vi "Read SubComponents.vi"(8 "error in (no error)":errorcluster, 11 "1553 Component in":refnum<class "1553 Component.lvclass">) -> (0 "error out":errorcluster, 2 "SubComponents":refnum<class "1553 SubComponent.lvclass">[](array[class]), 3 "1553 Component out":refnum<class "1553 Component.lvclass">)   [LabVIEW 2020, in "BCI-1553 API.lvlib" / "1553 Component.lvclass"]
doc: "Returns all the subcomponents being used by this component in a 1553 Session. After initialization, where applicable, all subcomponents are returned in this order:\n\n0: Bus Controller\n1-2: Remote Terminal(s)\n3: Bus Monitor\n\nThe order shifts towards index 0 if a subcomponent is not present during the initialization."
uses:
  1553 Component.lvclass
  1553 SubComponent/1553 SubComponent.lvclass
  1553 Component.lvclass/1553 Component.ctl
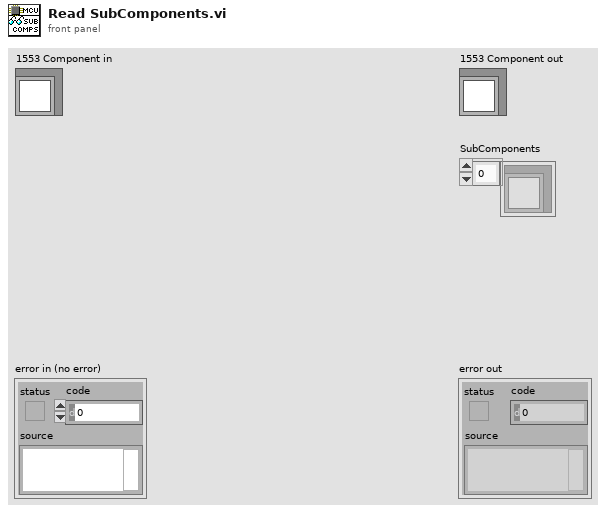
[diagram p1: front panel]
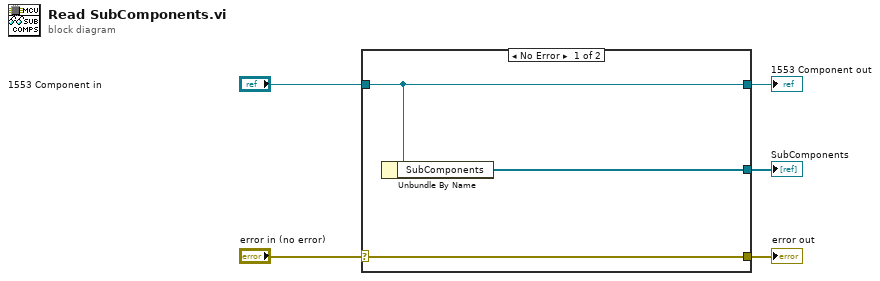
[diagram p0: block diagram]
diagram:
  n1 = case shown="No Error" "error in (no error)" {
    selector: "error in (no error)" -> [w8 w9]
    tunnel: [w8 w9] -> w4
    tunnel: [w7 w10] -> w2
    tunnel: "1553 Component in" -> [w7 w10]
    tunnel: [w6 _] -> w1
    frame No Error {
      n2 = Unbundle By Name(w7) -> ("SubComponents"=w6:refnum<class "1553 SubComponent.lvclass">[])
    }
    frame Error {
    }
  }
  "error out" <- w4
  "1553 Component out" <- w2
  "SubComponents" <- w1
